vi "Main.vi"() -> ()   [LabVIEW 2012]
doc: "Ce VI modèle est conçu pour le modèle de conception Gestionnaire de messages dans une file d'attente.\n\nLa boucle de gestion d'événements génère des messages en fonction des actions sur l'interface utilisateur.\n\nLa boucle de gestion de messages traite les messages générés par la boucle de gestion d'événements ou par d'autres messages. Les messages sont des valeurs chaîne ; il est donc facile d'ajouter de nouveaux messages à la structure condition Conditions de messages de la boucle de gestion de messages Chaque cluster Message peut en outre fournir une valeur optionnelle pour Données de message, un variant qui peut être converti aux données requises pour un message spécifique."
uses:
  controls/UI Data.ctl
  support/Message Queue/Message Queue.lvlib
  support/User Event - Stop/User Event - Stop.lvlib
panel:
  out "Affichage <À remplacer>":string
  in  "Faire action 2 <À remplacer>":bool
  in  "Faire action 1 <À remplacer>":bool
  in  "Bouton Stop":bool
  # "Ces commandes sont associées à des événements \"Valeur changée\" configurés dans la structure Événement du diagramme.\n\nRemplacez-les par les commandes nécessaires à votre application et reconfigurez la structure Événement."
  # "Ce VI modèle est conçu pour le modèle de conception Gestionnaire de messages dans une file d'attente.\n\nConsultez le diagramme pour en savoir plus sur comment utiliser ce modèle."
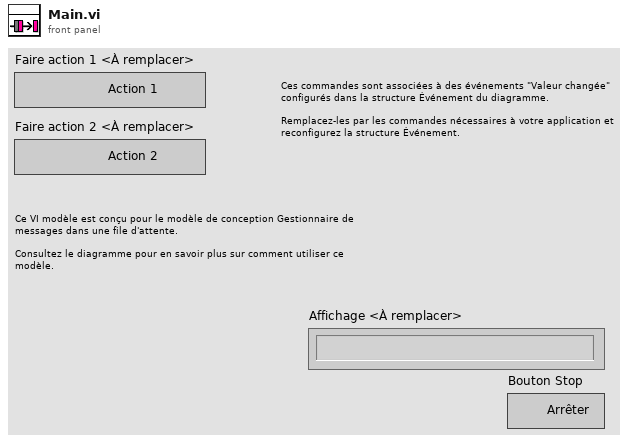
[diagram p1: front panel]
types:
  T1 = typedef "UI Data.ctl" = cluster{"Booléen <À remplacer>":bool, "Chaîne <À remplacer>":string, "Numérique <À remplacer>":dbl, "Réf. Action 1":refnum<vi>, "Réf. Action 2":refnum<vi>, "Réf. Affichage des données":refnum<vi>, "Réf. Bouton Stop":refnum<vi>}
  T2 = cluster{"état":bool, "code":i32, "source":string}
  T3 = typedef "Message Queue.lvlib/All Message Queues.ctl" = cluster{"IU":refnum<queue>}
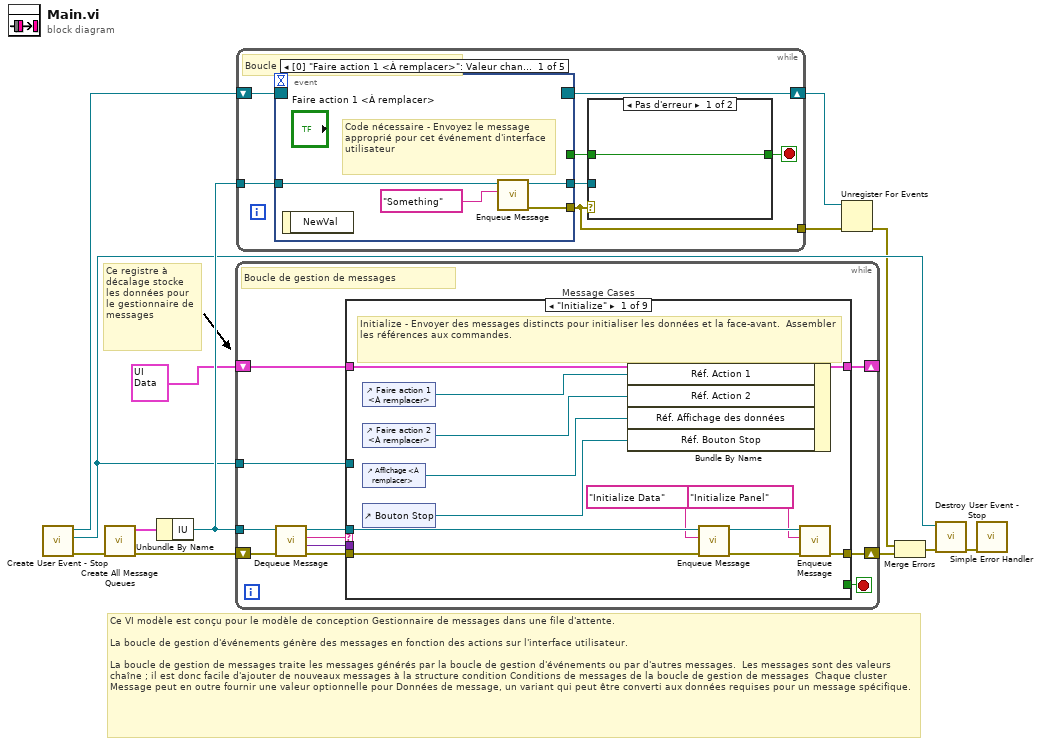
[diagram p0: block diagram]
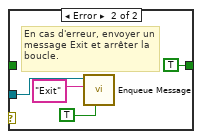
[diagram p2: hidden frame]
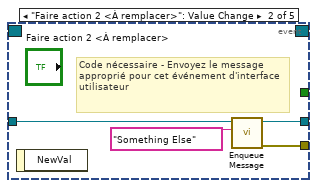
[diagram p3: hidden frame]
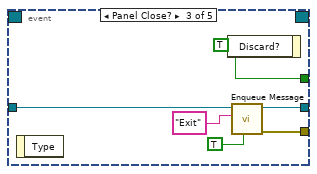
[diagram p4: hidden frame]
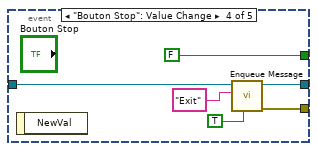
[diagram p5: hidden frame]
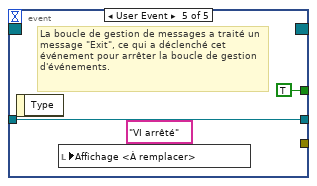
[diagram p6: hidden frame]
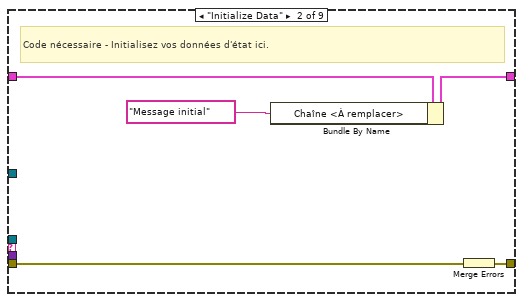
[diagram p7: hidden frame]
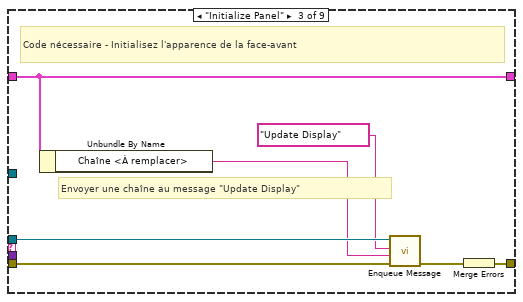
[diagram p8: hidden frame]
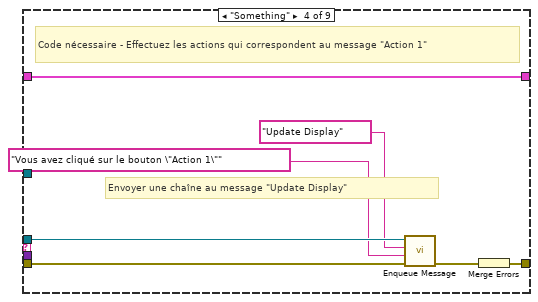
[diagram p9: hidden frame]
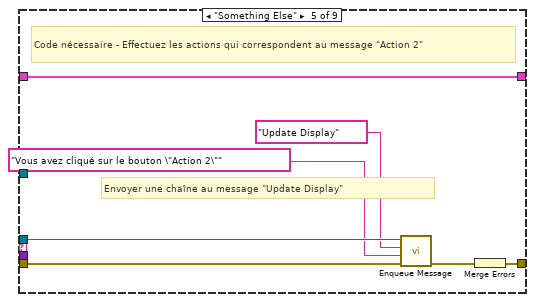
[diagram p10: hidden frame]
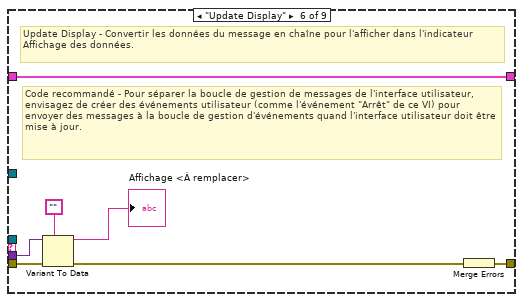
[diagram p11: hidden frame]
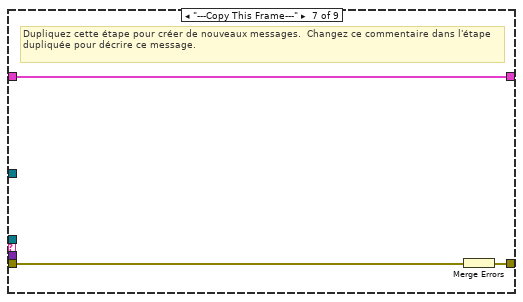
[diagram p12: hidden frame]
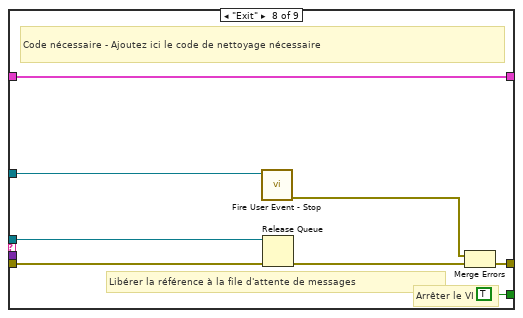
[diagram p13: hidden frame]
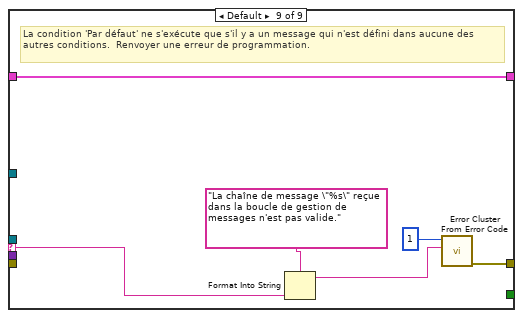
[diagram p14: hidden frame]
diagram:
  # "Ce VI modèle est conçu pour le modèle de conception Gestionnaire de messages dans une file d'attente.\n\nLa boucle de gestion d'événements génère des messages en fonction des actions sur l'interface utilisateur.\n\nLa boucle de gestion de messages traite les messages générés par la boucle de gestion d'événements ou par d'autres messages.  Les messages sont des valeurs chaîne ; il est donc facile d'ajouter de nouveaux messages à la structure condition Conditions de messages de la boucle de gestion de messages  Chaque cluster Message peut en outre fournir une valeur optionnelle pour Données de message, un variant qui peut être converti aux données requises pour un message spécifique."
  # "Ce registre à décalage stocke les données pour le gestionnaire de messages"
  n1 = call "Create User Event - Stop.vi"() -> ("error out"=w8:T2, "Événement utilisateur - Arrêt"=w5:refnum<user-event>, "Refnum Enregistrement à l'événement Arrêt"=w9:refnum<event-registration>)  [unwired: 9 in]
  n2 = call "Create All Message Queues.vi"("error in (no error)"=w8) -> ("error out"=w13:T2, "Files d'attente de messages en sortie"=w12:T3)  [unwired: 9 in]
  n3 = Unbundle By Name(w12) -> ("IU"=w10:refnum<queue>)
  n4 = while {
    tunnel: w10 -> [w14]
    shift-right: [w23] -> _
    shift-left: T1 {"Booléen <À remplacer>"=TRUE, "Chaîne <À remplacer>"="", "Numérique <À remplacer>"=0.0, "Réf. Action 1"=refnum, "Réf. Action 2"=refnum, "Réf. Affichage des données"=refnum, "Réf. Bouton Stop"=refnum} ("Data Cluster") -> [w24]
    tunnel: w5 -> [w20]
    shift-right: [w21] -> w11
    shift-left: w13 -> [w19]
    stop <- w22 stop-if-true
    # "Boucle de gestion de messages"
    n5 = call "Dequeue Message.vi"("error in (no error)"=w19, "File d'attente de messages"=w14) -> ("error out"=w18:T2, "Données de message"=w16:variant, "Message"=w17:string, "File d'attente de message dup."=w15:refnum<queue>)  [unwired: 6 in]
    n6 = case "Message Cases" shown="\"Initialize\"" w17 {
      selector: w17 -> [_ _ _ _ _ _ _ _ w85]
      tunnel: w15 -> [w33 _ w46 w52 w59 _ _ w81 _]
      tunnel: w18 -> [w36 w42 w47 w54 w61 w68 w73 w76 _]
      tunnel: [w37 w38 w48 w55 w62 w69 w71 w77 w83] -> w21
      tunnel: w24 -> [w30 w41 w49 w56 w63 w70 w72 w80 w87]
      tunnel: [w29 w40 w49 w56 w63 w70 w72 w80 w87] -> w23
      tunnel: [_ _ _ _ _ _ _ TRUE _] -> w22
      tunnel: w16 -> [_ _ _ _ _ w67 _ _ _]
      tunnel: w20 -> [_ _ _ _ _ _ _ w75 _]
      frame "Initialize" {
        # "Initialize - Envoyer des messages distincts pour initialiser les données et la face-avant.  Assembler les références aux commandes."
        n7 = control-ref of="Faire action 1 <À remplacer>"() -> (w28:refnum<vi>)
        n8 = control-ref of="Faire action 2 <À remplacer>"() -> (w27:refnum<vi>)
        n9 = control-ref of="Affichage <À remplacer>"() -> (w26:refnum<vi>)
        n10 = control-ref of="Bouton Stop"() -> (w25:refnum<vi>)
        n11 = Bundle By Name(cluster=w30, "Réf. Action 1"=w28, "Réf. Action 2"=w27, "Réf. Affichage des données"=w26, "Réf. Bouton Stop"=w25) -> (w29:T1)
        n12 = call "Enqueue Message.vi"("error in (no error)"=w36, "Message"="Initialize Data", "File d'attente de messages"=w33) -> ("error out"=w35:T2, "File d'attente de message dup."=w34:refnum<queue>)  [unwired: 7 in]
        n13 = call "Enqueue Message.vi"("error in (no error)"=w35, "Message"="Initialize Panel", "File d'attente de messages"=w34) -> ("error out"=w37:T2)  [unwired: 7 in, 1 out]
      }
      frame "Initialize Data" {
        # "Code nécessaire - Initialisez vos données d'état ici."
        n14 = Bundle By Name(cluster=w41, "Chaîne <À remplacer>"="Message initial" ("Initial Message")) -> (w40:T1)
        n15 = Merge Errors(w42) -> (w38:errorcluster)
      }
      frame "Initialize Panel" {
        # "Envoyer une chaîne au message \"Update Display\""
        # "Code nécessaire - Initialisez l'apparence de la face-avant"
        n16 = Unbundle By Name(w49) -> ("Chaîne <À remplacer>"=w43:string)
        n17 = call "Enqueue Message.vi"("error in (no error)"=w47, "Données de message"=w43, "Message"="Update Display", "File d'attente de messages"=w46) -> ("error out"=w45:T2)  [unwired: 6 in, 1 out]
        n18 = Merge Errors(w45) -> (w48:errorcluster)
      }
      frame "Something" {
        # "Envoyer une chaîne au message \"Update Display\""
        # "Code nécessaire - Effectuez les actions qui correspondent au message \"Action 1\""
        n19 = call "Enqueue Message.vi"("error in (no error)"=w54, "Données de message"="Vous avez cliqué sur le bouton \"Action 1\"" ("\"Do Something\" button pressed"), "Message"="Update Display", "File d'attente de messages"=w52) -> ("error out"=w53:T2)  [unwired: 6 in, 1 out]
        n20 = Merge Errors(w53) -> (w55:errorcluster)
      }
      frame "Something Else" {
        # "Envoyer une chaîne au message \"Update Display\""
        # "Code nécessaire - Effectuez les actions qui correspondent au message \"Action 2\""
        n21 = call "Enqueue Message.vi"("error in (no error)"=w61, "Données de message"="Vous avez cliqué sur le bouton \"Action 2\"" ("\"Do Something Else\" button pressed"), "Message"="Update Display", "File d'attente de messages"=w59) -> ("error out"=w60:T2)  [unwired: 6 in, 1 out]
        n22 = Merge Errors(w60) -> (w62:errorcluster)
      }
      frame "Update Display" {
        # "Code recommandé - Pour séparer la boucle de gestion de messages de l'interface utilisateur, envisagez de créer des événements utilisateur (comme l'événement \"Arrêt\" de ce VI) pour envoyer des messages à la boucle de gestion d'événements quand l'interface utilisateur doit être mise à jour."
        # "Update Display - Convertir les données du message en chaîne pour l'afficher dans l'indicateur Affichage des données."
        n23 = Variant To Data(error in=w68, type="", Variant=w67) -> (data=→"Affichage <À remplacer>":string, error out=w65:errorcluster)
        n24 = Merge Errors(w65) -> (w69:errorcluster)
      }
      frame "---Copy This Frame---" {
        # "Dupliquez cette étape pour créer de nouveaux messages.  Changez ce commentaire dans l'étape dupliquée pour décrire ce message."
        n25 = Merge Errors(w73) -> (w71:errorcluster)
      }
      frame "Exit" {
        # "Arrêter le VI"
        # "Libérer la référence à la file d'attente de messages"
        # "Code nécessaire - Ajoutez ici le code de nettoyage nécessaire"
        n26 = call "Fire User Event - Stop.vi"("Événement utilisateur - Arrêt"=w75) -> ("error out"=w74:T2)  [unwired: 10 in]
        n27 = Release Queue(queue=w81, error in (no error)=w76) -> (error out=w78:errorcluster)  [unwired: 1 in, 2 out]
        n28 = Merge Errors(w74, w78) -> (w77:errorcluster)
      }
      frame Default {
        # "La condition 'Par défaut' ne s'exécute que s'il y a un message qui n'est défini dans aucune des autres conditions.  Renvoyer une erreur de programmation."
        n29 = Format Into String(format string="La chaîne de message \"%s\" reçue dans la boucle de gestion de messages n'est pas valide." ("Unknown Message Error Text"), w85) -> (resulting string=w82:string)  [unwired: 2 in, 1 out]
        n30 = call <vilib>:"Error Cluster From Error Code.vi"("error message (\"\")"=w82, "error code (0)"=1) -> ("error out"=w83:errorcluster)  [unwired: 7 in]
      }
    }
  }
  n31 = while {
    tunnel: w10 -> [w94]
    tunnel: [w90] -> w3
    shift-right: [w88] -> w2
    shift-left: w9 -> [w89]
    stop <- w92 stop-if-true
    # "Boucle de gestion d'événements"
    n32 = event shown="[0] \"Faire action 1 <À remplacer>\": Valeur changée" {
      selector: w89 -> [_ _ _ _ _]
      dyn-events: [_ _ _ _ _] -> w88
      timeout: _ -> [_ _ _ _ _]
      tunnel: [_ _ w113 FALSE ("Discard?") TRUE ("Discard?")] -> w93
      tunnel: w94 -> [w103 w107 w112 w119 w122]
      tunnel: [w102 w105 w111 w118 _] -> w90
      tunnel: [w101 w106 w110 w116 w122] -> w91
      event "Faire action 1 <À remplacer>": Value Change {
        # "Code nécessaire - Envoyez le message approprié pour cet événement d'interface utilisateur"
        n33 = event-data() -> ()  [unwired: 1 in, 1 out]
        n34 = call "Enqueue Message.vi"("Message"="Something", "File d'attente de messages"=w103) -> ("error out"=w102:T2, "File d'attente de message dup."=w101:refnum<queue>)  [unwired: 8 in]
      }
      event "Faire action 2 <À remplacer>": Value Change {
        # "Code nécessaire - Envoyez le message approprié pour cet événement d'interface utilisateur"
        n35 = event-data() -> ()  [unwired: 1 in, 1 out]
        n36 = call "Enqueue Message.vi"("Message"="Something Else", "File d'attente de messages"=w107) -> ("error out"=w105:T2, "File d'attente de message dup."=w106:refnum<queue>)  [unwired: 8 in]
      }
      event Panel Close? {
        w113 = TRUE ("Discard?")
        n37 = event-data() -> ()  [unwired: 1 in, 1 out]
        n38 = event-data("Discard?"=w113) -> ()  [unwired: 1 in, 1 out]
        n39 = call "Enqueue Message.vi"("Message prioritaire ? (F)"=TRUE ("Priority Message? (F)"), "Message"="Exit", "File d'attente de messages"=w112) -> ("error out"=w111:T2, "File d'attente de message dup."=w110:refnum<queue>)  [unwired: 7 in]
      }
      event "Bouton Stop": Value Change {
        n40 = event-data() -> ()  [unwired: 1 in, 1 out]
        n41 = call "Enqueue Message.vi"("Message prioritaire ? (F)"=TRUE ("Priority Message? (F)"), "Message"="Exit", "File d'attente de messages"=w119) -> ("error out"=w118:T2, "File d'attente de message dup."=w116:refnum<queue>)  [unwired: 7 in]
      }
      event User Event {
        # "La boucle de gestion de messages a traité un message \"Exit\", ce qui a déclenché cet événement pour arrêter la boucle de gestion d'événements."
        n42 = event-data() -> ()  [unwired: 1 in, 1 out]
        n43 = local write "Affichage <À remplacer>"("VI arrêté" ("VI Stopped")) -> ()
      }
    }
    n44 = case shown="Pas d'erreur" w90 {
      tunnel: [w95 TRUE ("Discard?")] -> w92
      tunnel: w93 -> [w95 _]
      tunnel: w91 -> [_ w98]
      frame No Error {
      }
      frame Error {
        # "En cas d'erreur, envoyer un message Exit et arrêter la boucle."
        n45 = call "Enqueue Message.vi"("Message prioritaire ? (F)"=TRUE ("Priority Message? (F)"), "Message"="Exit", "File d'attente de messages"=w98) -> ()  [unwired: 7 in, 2 out]
      }
    }
  }
  n46 = Unregister For Events(event registration refnum=w2, error in=w3) -> (error out=w4:errorcluster)
  n47 = Merge Errors(w4, w11) -> (w6:errorcluster)
  n48 = call "Destroy User Event - Stop.vi"("error in (no error)"=w6, "Événement utilisateur - Arrêt"=w5) -> ("error out"=w7:T2)  [unwired: 9 in]
  n49 = call <vilib>:"Simple Error Handler.vi"("error in (no error)"=w7) -> ()  [unwired: 4 in, 5 out]
